vi "Variant_BuildClusterFromElementArray.vi"(9 "name":string, 10 "Elements":variant[](array[variant])) -> (3 "Cluster":variant)   [LabVIEW 2022 SP3, in "hse-misc.lvlib"]
doc: "From the LabVIEW Open Source project DataManipulation library v1.4.0 by Francois Normandin (https://github.com/LabVIEW-Open-Source/DataManipulation).\n\n____\nHAMPEL SOFTWARE ENGINEERING v3.8.0 (2023-12-18 14:41)"
uses:
  hse-misc.lvlib
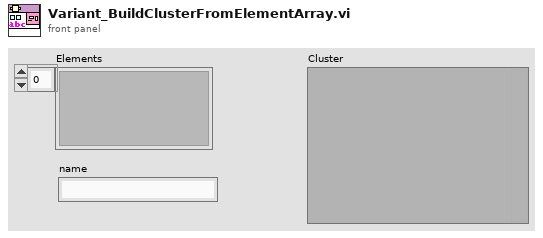
[diagram p1: front panel]
types:
  T1 = typedef "Type Descriptor I16 Array.ctl" = T2[]
  T2 = typedef "Type Descriptor I16.ctl" = i16
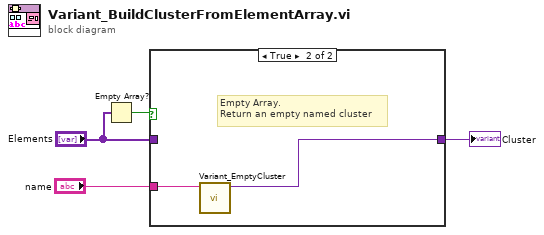
[diagram p0: block diagram]
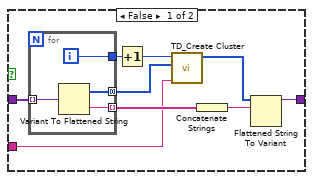
[diagram p2: hidden frame]
diagram:
  n1 = Empty Array?(array="Elements") -> (empty?=w1:bool)
  n2 = case shown="True" w1 {
    tunnel: [w11 w18] -> w3
    tunnel: "name" -> [w8 w19]
    tunnel: "Elements" -> [w5 _]
    frame False {
      n3 = for {
        tunnel: w5 -> [w17] mode=indexing
        tunnel: [w16] -> w6 mode=concatenating
        tunnel: [w15] -> w12 mode=indexing
        tunnel: [w14] -> w10
        i -> [w14]
        n4 = Variant To Flattened String(Variant=w17) -> (data string=w15:string, 1:w16:i16[])
      }
      n5 = Increment(x=w10) -> (x+1=w9:i32)
      n6 = call <vilib>:"TD_Create Cluster.vi"("Name"=w8, "Concatenated Elts"=w6, "N Elts"=w9) -> ("ClusterTD"=w7:T1)  [unwired: 8 in]
      n7 = Concatenate Strings(w12) -> (w13:string)
      n8 = Flattened String To Variant(6:w13, 7:w7) -> (3:w11:variant)  [unwired: 1 in, 1 out]
    }
    frame True {
      # "Empty Array.\nReturn an empty named cluster"
      n9 = call "Variant_EmptyCluster.vi"("Cluster Name"=w19) -> ("Empty Cluster"=w18:variant)  [unwired: 10 in]
    }
  }
  "Cluster" <- w3
